vi "MainV1.vi"() -> ()   [LabVIEW 2015]
uses:
  <vilib>/userdefined/High Color/IMAQdx.ctl
  <vilib>/MakerHub/LINX/Public/Peripherals/Digital/Digital Write 1 Chan.vi
  <vilib>/MakerHub/LINX/Public/Peripherals/Digital/Digital Read 1 Chan.vi
  <vilib>/MakerHub/LINX/Public/Peripherals/Digital/Digital Write N Chans.vi
  <vilib>/MakerHub/LINX/Public/Peripherals/Digital/Digital Read N Chans.vi
  <vilib>/MakerHub/LINX/Private/Local IO/LinxDigitalWrite.vi
  <vilib>/MakerHub/LINX/Public/Utilities/Check Channel.vi
  <vilib>/MakerHub/LINX/Private/Local IO/LinxDigitalRead.vi
  <vilib>/MakerHub/LINX/Public/Utilities/Open Serial.vi
  <vilib>/MakerHub/LINX/Private/Utilties/Generate Error.vi
  <vilib>/MakerHub/LINX/LMH-LINX.lvlib
  <vilib>/vision/driver/NI_Vision_Acquisition_Software.lvlib
panel:
  out "DI Value":bool
  in  "Capture":bool
  out "Image Original":T1(plugin-control)
  out "PROCESS STATE":T2(ring)
  out "Arduino Error Out":errorcluster
  in  "Process Stop Button":bool
  in  "Play Button":bool
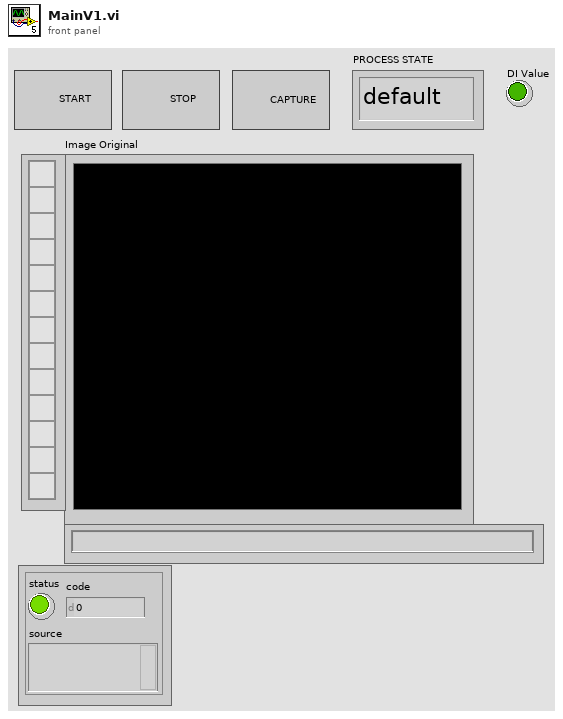
[diagram p1: front panel]
types:
  T1 = typedef "IMAQ Image.ctl" = refnum<image>
  T2 = enum16{"default", "Initial", "Conveyor", "Vision", "Polish", "ShiftJig", "Stop", ""}
  T3 = typedef "IMAQdx.ctl" = refnum<k21>
  T4 = typedef "Image Type" = u32
  T5 = typedef "LMH-LINX.lvlib/LINX Ref.ctl" = cluster{"IO":T6, "Interface":T7, "LINX Device Config":T8}
  T6 = typedef "LMH-LINX.lvlib/Platform.ctl" = enum16{"Remote", "Local"}
  T7 = typedef "LMH-LINX.lvlib/Interface.ctl" = enum16{"Serial", "TCP"}
  T8 = typedef "LMH-LINX.lvlib/Device.lvlib/LINX Device Config.ctl" = cluster{"Interface":T7, "COM Port":refnum<visa-resource-name>, "TCP Configuration":T9, "Device Family":u8, "Device ID":u8, "Device Name":string, "TCP Ref":refnum<k5>, "Channels":T10}
  T9 = typedef "LMH-LINX.lvlib/Device.lvlib/TCP Config.ctl" = cluster{"IP Address":string, "Port":u16}
  T10 = typedef "LMH-LINX.lvlib/Channels.ctl" = cluster{"DI":u8[], "DO":u8[], "AI":u8[], "AO":u8[], "PWM":u8[], "QE":u8[], "UART":u8[], "I2C 2":u8[], "SPI":u8[], "CAN":u8[], "Servo":u8[], "AI Ref (V)":dbl, "AI Resolution (Bits)":u8, "AO Ref (V)":dbl, "AO Resolution (Bits)":u8}
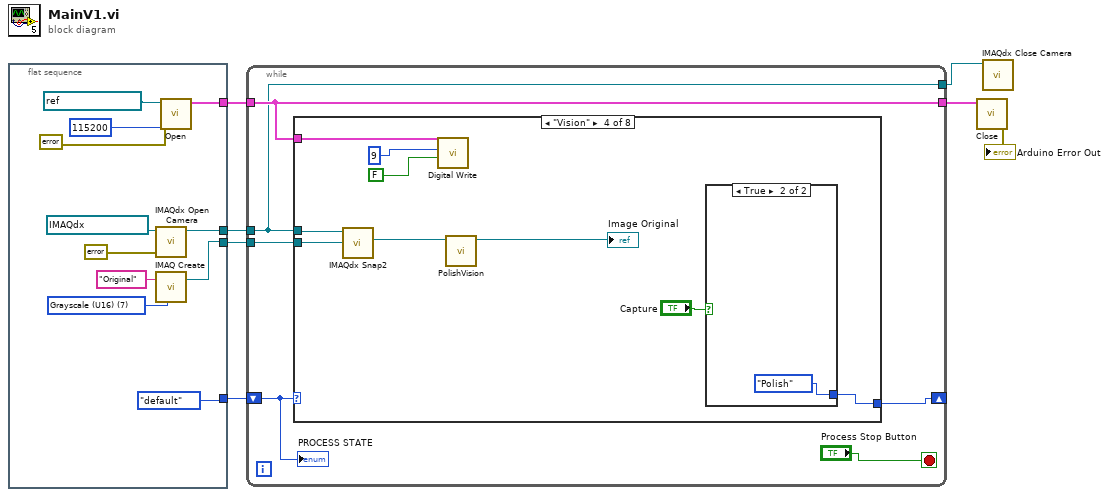
[diagram p0: block diagram]
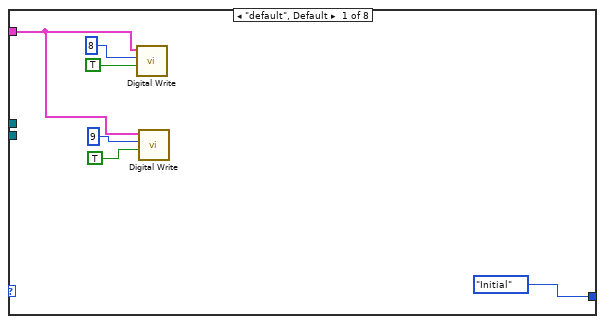
[diagram p2: hidden frame]
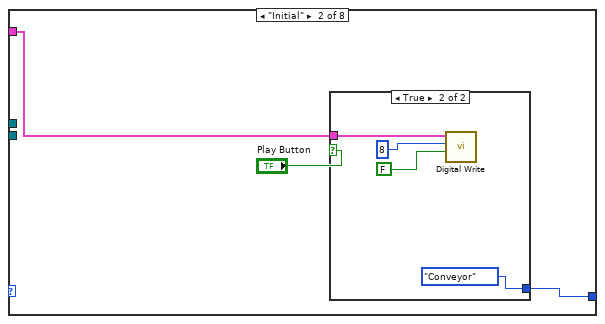
[diagram p3: hidden frame]
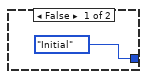
[diagram p4: hidden frame]
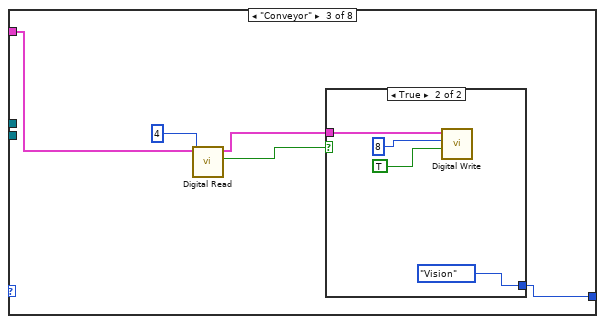
[diagram p5: hidden frame]
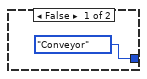
[diagram p6: hidden frame]
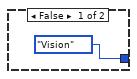
[diagram p7: hidden frame]
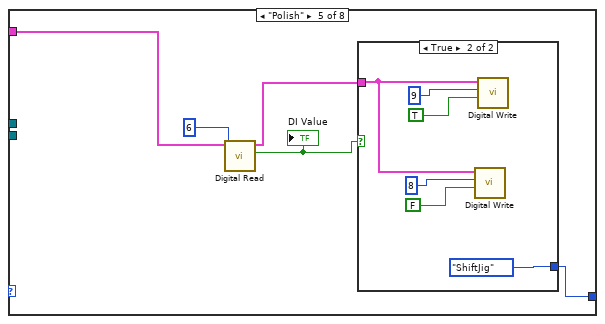
[diagram p8: hidden frame]
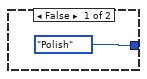
[diagram p9: hidden frame]
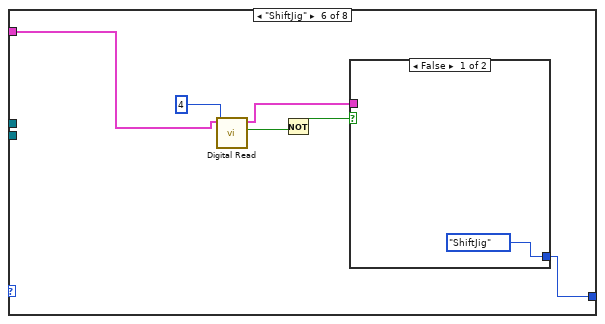
[diagram p10: hidden frame]
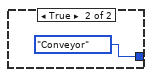
[diagram p11: hidden frame]
diagram:
  n1 = flat-sequence {
    tunnel: [T2."default"] -> w7
    tunnel: [w15] -> w6
    tunnel: [w9] -> w3
    tunnel: [w8] -> w2
    frame #0 {
      w12 = T4 7 items=["Grayscale (U8)", "Grayscale (I16)", "Grayscale (SGL)", "Complex (CSG)", "RGB (U32)", "HSL (U32)", "RGB (U64)", "Grayscale (U16)"] ("Image Type")
      n2 = call <vilib>:"IMAQdx Open Camera.vi"("error in"=errorcluster {"status"=FALSE, "code"=0, "source"=""}, "Session In"=T3 "acA1920-25gc") -> ("Session Out"=w9:T3)  [unwired: 8 in, 1 out]
      n3 = call "IMAQ Create"("Image Name"="Original", "Image Type"=w12) -> ("New Image"=w8:T1)  [unwired: 3 in, 1 out]
      n4 = call-poly <vilib>:"Open.vi"("Error In"=errorcluster {"status"=FALSE, "code"=0, "source"=""}, "Baud Rate Override"=u32 115200, "Serial Port"=refnum<visa-resource-name> "COM4") -> ("LINX Resource"=w15:T5)  [unwired: 6 in, 2 out]
    }
  }
  n5 = while {
    tunnel: w6 -> [w21]
    shift-right: [w23] -> _
    shift-left: w7 -> [w24]
    tunnel: [w21] -> w4
    tunnel: w3 -> [w19]
    tunnel: w2 -> [w20]
    tunnel: [w19] -> w1
    stop <- "Process Stop Button" stop-if-true
    n6 = case shown="\"Vision\"" w24 {
      tunnel: w21 -> [w25 w31 w42 w55 w62 w74 _ _]
      tunnel: [T2."Initial" w32 w41 w54 w61 w72 _ _] -> w23
      tunnel: w19 -> [_ _ _ w53 _ _ _ _]
      tunnel: w20 -> [_ _ _ w52 _ _ _ _]
      frame "default", Default {
        n7 = call-poly <vilib>:"Digital Write.vi"("Output Value"=TRUE, "DO Channel"=u8 8, "LINX Resource"=w25) -> ()  [unwired: 7 in, 2 out]
        n8 = call-poly <vilib>:"Digital Write.vi"("Output Value"=TRUE, "DO Channel"=u8 9, "LINX Resource"=w25) -> ()  [unwired: 7 in, 2 out]
      }
      frame "Initial" {
        n9 = case shown="True" "Play Button" {
          tunnel: [T2."Initial" T2."Conveyor"] -> w32
          tunnel: w31 -> [_ w35]
          frame False {
          }
          frame True {
            n10 = call-poly <vilib>:"Digital Write.vi"("Output Value"=FALSE, "DO Channel"=u8 8, "LINX Resource"=w35) -> ()  [unwired: 7 in, 2 out]
          }
        }
      }
      frame "Conveyor" {
        n11 = call-poly <vilib>:"Digital Read.vi"("DI Channel"=u8 4, "LINX Resource"=w42) -> ("DI Value"=w39:bool, "LINX Resource"=w40:T5)  [unwired: 7 in, 1 out]
        n12 = case shown="True" w39 {
          tunnel: [T2."Conveyor" T2."Vision"] -> w41
          tunnel: w40 -> [_ w45]
          frame False {
          }
          frame True {
            n13 = call-poly <vilib>:"Digital Write.vi"("Output Value"=TRUE, "DO Channel"=u8 8, "LINX Resource"=w45) -> ()  [unwired: 7 in, 2 out]
          }
        }
      }
      frame "Vision" {
        n14 = call <vilib>:"IMAQdx Snap2.vi"("Image In"=w52, "Session In"=w53) -> ("Image Out"=w51:T1)  [unwired: 7 in, 2 out]
        n15 = call-poly <vilib>:"Digital Write.vi"("Output Value"=FALSE, "DO Channel"=u8 9, "LINX Resource"=w55) -> ()  [unwired: 7 in, 2 out]
        n16 = call "PolishVision.vi"("Refnum in"=w51) -> ("Refnum out"=→"Image Original":T1)  [unwired: 10 in]
        n17 = case shown="True" "Capture" {
          tunnel: [T2."Vision" T2."Polish"] -> w54
          frame False {
          }
          frame True {
          }
        }
      }
      frame "Polish" {
        n18 = call-poly <vilib>:"Digital Read.vi"("DI Channel"=u8 6, "LINX Resource"=w62) -> ("DI Value"=w60:bool, "LINX Resource"=w63:T5)  [unwired: 7 in, 1 out]
        "DI Value" <- w60
        n19 = case shown="True" w60 {
          tunnel: [T2."Polish" T2."ShiftJig"] -> w61
          tunnel: w63 -> [_ w66]
          frame False {
          }
          frame True {
            n20 = call-poly <vilib>:"Digital Write.vi"("Output Value"=FALSE, "DO Channel"=u8 8, "LINX Resource"=w66) -> ()  [unwired: 7 in, 2 out]
            n21 = call-poly <vilib>:"Digital Write.vi"("Output Value"=TRUE, "DO Channel"=u8 9, "LINX Resource"=w66) -> ()  [unwired: 7 in, 2 out]
          }
        }
      }
      frame "ShiftJig" {
        n22 = call-poly <vilib>:"Digital Read.vi"("DI Channel"=u8 4, "LINX Resource"=w74) -> ("DI Value"=w75:bool, "LINX Resource"=w76:T5)  [unwired: 7 in, 1 out]
        n23 = Not(x=w75) -> (.not. x?=w73:bool)
        n24 = case shown="False" w73 {
          tunnel: [T2."ShiftJig" T2."Conveyor"] -> w72
          tunnel: w76 -> [_ _]
          frame False {
          }
          frame True {
          }
        }
      }
      frame "Stop" {
      }
      frame "" {
      }
    }
    "PROCESS STATE" <- w24
  }
  n25 = call <vilib>:"Close.vi"("LINX Resource"=w4) -> ("Error Out"=→"Arduino Error Out":errorcluster)  [unwired: 10 in]
  n26 = call <vilib>:"IMAQdx Close Camera.vi"("Session In"=w1) -> ()  [unwired: 10 in, 1 out]
